vi "NF90 stop.vi"(2 "Stop":T1, 3 "port number":refnum<visa-resource-name>) -> ()   [LabVIEW 2015]
uses:
  Kill.ctl
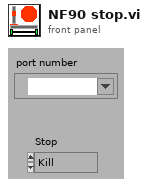
[diagram p1: front panel]
types:
  T1 = typedef "Kill.ctl" = enum16{"Kill", "Decelerate"}
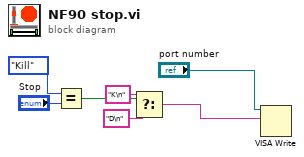
[diagram p0: block diagram]
diagram:
  n1 = Equal?(x=enum16{"Kill", "Decelerate"}."Kill", y="Stop") -> (x = y?=w3:bool)
  n2 = Select(t="K\n" ("string to write"), s=w3, f="D\n" ("string to write")) -> (s? t:f=w1:string)
  n3 = VISA Write(VISA resource name="port number", write buffer=w1) -> ()  [unwired: 1 in, 3 out]
